vi "Get DDG Gate Time.vi"(8 "error in (no error)":errorcluster, 10 "puiWidth":cluster{}, 11 "puiDelay":cluster{}) -> (0 "error out":errorcluster, 1 "function return":u32, 2 "puiWidth out":cluster{}, 3 "puiDelay out":cluster{})   [LabVIEW 2014, in "atmcd32d.lvlib"]
doc: "unsigned int WINAPI GetDDGGateTime(at_u64 * puiDelay, at_u64 * puiWidth);"
uses:
  atmcd32d.lvlib
  atmcd32d.dll
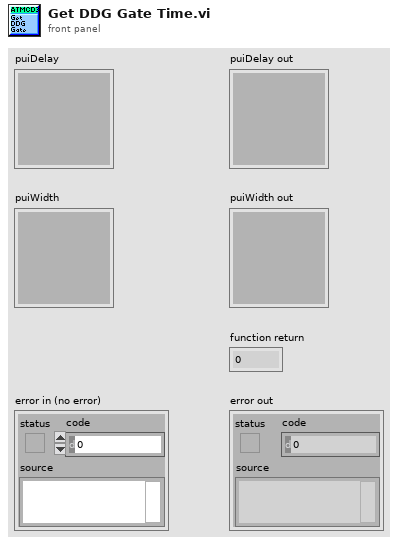
[diagram p1: front panel]
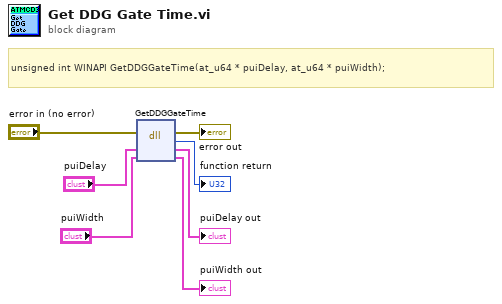
[diagram p0: block diagram]
diagram:
  # "unsigned int WINAPI GetDDGGateTime(at_u64 * puiDelay, at_u64 * puiWidth);"
  n1 = dll-call lib="C:/Users/Bakir/Documents/Lambda2-Testing/lib/Andorlib/atmcd32d.*" fn="GetDDGGateTime"(error in="error in (no error)", "puiDelay"="puiDelay", "puiWidth"="puiWidth") -> (error out=→"error out":errorcluster, →"function return":u32, "puiDelay"=→"puiDelay out":cluster{}, "puiWidth"=→"puiWidth out":cluster{})  [unwired: 2 in, 1 out]
